vi "Edit 1.vi"() -> ()   [LabVIEW 2021]
panel:
  in  "Tab Control":enum32{"Page 1", "Page 2"}(tab)
  out "Bill":dbl
  out "discount":string
  out "Price per 1kg (Rs.)":dbl
  out "price 4":dbl
  out "price 3":dbl
  out "price 2":dbl
  out "Vegetables":dbl
  in  "Carrot":bool
  in  "quantity 5":dbl
  in  "Cabege":bool
  in  "quantity 4":dbl
  in  "Bringle":bool
  in  "quantity 3":dbl
  in  "Beans":bool
  in  "quantity 2":dbl
  in  "Leeks":bool
  in  "Quantities(kg)":dbl
  out "Total Bill":dbl
  in  "Banana":bool
  out "Fruits":dbl
  in  "Apple":bool
  out "price 6":dbl
  in  "quantity 6":dbl
  in  "Orange":bool
  out "price 7":dbl
  in  "quantity 7":dbl
  in  "Graps":bool
  out "price 8":dbl
  in  "quantity 8":dbl
  in  "Papaya":bool
  in  "quantity 9":dbl
  out "Price per 1kg 2":dbl
  in  "Quantities 2":dbl
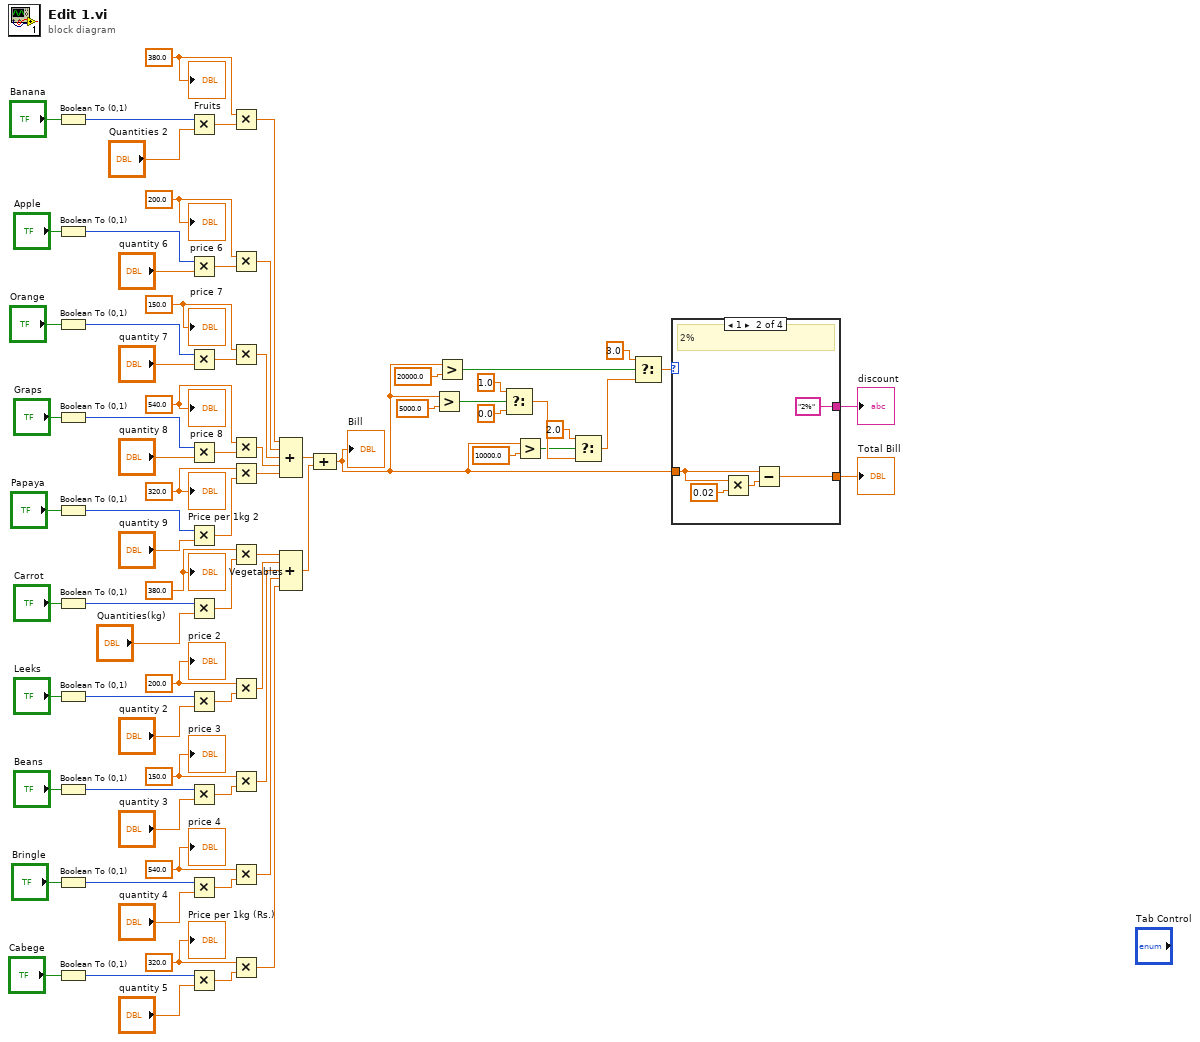
[diagram p0: block diagram]
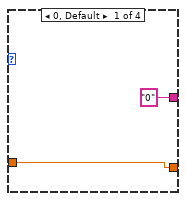
[diagram p2: hidden frame]
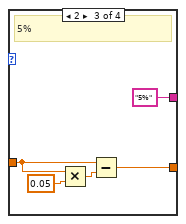
[diagram p3: hidden frame]
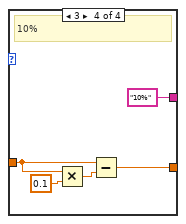
[diagram p4: hidden frame]
diagram:
  w52 = 320.0 ("price")
  w59 = 540.0 ("price")
  w62 = 150.0 ("price")
  w69 = 200.0 ("price")
  w72 = 380.0 ("price")
  w22 = 320.0 ("price")
  w29 = 540.0 ("price")
  w32 = 150.0 ("price")
  w39 = 200.0 ("price")
  w42 = 380.0 ("price")
  n1 = Boolean To (0,1)(Boolean="Banana") -> (0, 1=w74:i16)
  n2 = Boolean To (0,1)(Boolean="Apple") -> (0, 1=w67:i16)
  n3 = Boolean To (0,1)(Boolean="Orange") -> (0, 1=w64:i16)
  n4 = Boolean To (0,1)(Boolean="Graps") -> (0, 1=w57:i16)
  n5 = Boolean To (0,1)(Boolean="Papaya") -> (0, 1=w54:i16)
  n6 = Boolean To (0,1)(Boolean="Carrot") -> (0, 1=w44:i16)
  n7 = Boolean To (0,1)(Boolean="Leeks") -> (0, 1=w37:i16)
  n8 = Boolean To (0,1)(Boolean="Beans") -> (0, 1=w34:i16)
  n9 = Boolean To (0,1)(Boolean="Bringle") -> (0, 1=w27:i16)
  n10 = Boolean To (0,1)(Boolean="Cabege") -> (0, 1=w24:i16)
  n11 = Multiply(x=w74, y="Quantities 2") -> (x*y=w71:dbl)
  n12 = Multiply(x=w67, y="quantity 6") -> (x*y=w70:dbl)
  n13 = Multiply(x=w64, y="quantity 7") -> (x*y=w61:dbl)
  n14 = Multiply(x=w57, y="quantity 8") -> (x*y=w60:dbl)
  n15 = Multiply(x=w54, y="quantity 9") -> (x*y=w51:dbl)
  n16 = Multiply(x=w44, y="Quantities(kg)") -> (x*y=w41:dbl)
  n17 = Multiply(x=w37, y="quantity 2") -> (x*y=w40:dbl)
  n18 = Multiply(x=w34, y="quantity 3") -> (x*y=w31:dbl)
  n19 = Multiply(x=w27, y="quantity 4") -> (x*y=w30:dbl)
  n20 = Multiply(x=w24, y="quantity 5") -> (x*y=w21:dbl)
  n21 = Multiply(x=w72, y=w71) -> (x*y=w50:dbl)
  n22 = Multiply(x=w69, y=w70) -> (x*y=w49:dbl)
  n23 = Multiply(x=w62, y=w61) -> (x*y=w48:dbl)
  n24 = Multiply(x=w59, y=w60) -> (x*y=w47:dbl)
  n25 = Multiply(x=w52, y=w51) -> (x*y=w46:dbl)
  n26 = Multiply(x=w42, y=w41) -> (x*y=w20:dbl)
  n27 = Multiply(x=w39, y=w40) -> (x*y=w19:dbl)
  n28 = Multiply(x=w32, y=w31) -> (x*y=w18:dbl)
  n29 = Multiply(x=w29, y=w30) -> (x*y=w17:dbl)
  n30 = Multiply(x=w22, y=w21) -> (x*y=w16:dbl)
  n31 = Compound Arithmetic op=ADD(w50, w49, w48, w47, w46) -> (w77:dbl)
  n32 = Compound Arithmetic op=ADD(w20, w19, w18, w17, w16) -> (w76:dbl)
  n33 = Compound Arithmetic op=ADD(w77, w76) -> (w78:dbl)
  "Bill" <- w78
  n34 = Greater?(x=w78, y=5000.0) -> (0:w4:bool)
  n35 = Greater?(x=w78, y=20000.0) -> (0:w2:bool)
  n36 = Select(t=1.0, s=w4, f=0.0) -> (s? t:f=w8:dbl)
  n37 = Greater?(x=w78, y=10000.0) -> (0:w3:bool)
  n38 = Select(t=2.0, s=w3, f=w8) -> (s? t:f=w7:dbl)
  n39 = Select(t=3.0, s=w2, f=w7) -> (s? t:f=w6:dbl)
  n40 = case shown="1" w6 {
    tunnel: [w80 w84 w87 w92] -> w1
    tunnel: w78 -> [w80 w82 w88 w93]
    tunnel: ["0" ("discount") "2%" ("discount") "5%" ("discount") "10%" ("discount")] -> w5
    frame 0, Default {
    }
    frame 1 {
      # "2%"
      n41 = Multiply(x=w82, y=0.02) -> (x*y=w83:dbl)
      n42 = Subtract(x=w82, y=w83) -> (x-y=w84:dbl)
    }
    frame 2 {
      # "5%"
      n43 = Multiply(x=w88, y=0.05) -> (x*y=w89:dbl)
      n44 = Subtract(x=w88, y=w89) -> (x-y=w87:dbl)
    }
    frame 3 {
      # "10%"
      n45 = Multiply(x=w93, y=0.1) -> (x*y=w94:dbl)
      n46 = Subtract(x=w93, y=w94) -> (x-y=w92:dbl)
    }
  }
  "Total Bill" <- w1
  "discount" <- w5
  "Vegetables" <- w42
  "price 2" <- w39
  "price 3" <- w32
  "price 4" <- w29
  "Price per 1kg (Rs.)" <- w22
  "Fruits" <- w72
  "price 6" <- w69
  "price 7" <- w62
  "price 8" <- w59
  "Price per 1kg 2" <- w52
